vi "HB_ReadAISingleChannel.vi"(8 "error in (no error)":errorcluster, 10 "AI Channel":u8 max=7 step=1, 11 "HBDeviceRef":T1) -> (0 "error out":errorcluster, 1 "Raw Voltage":u32, 2 "Scaled Voltage":dbl, 3 "HBDeviceRef":T1)   [LabVIEW 2016]
uses:
  <vilib>/Rock Robotics/WPI/SerialPort/WPI_SerialPortRef.ctl
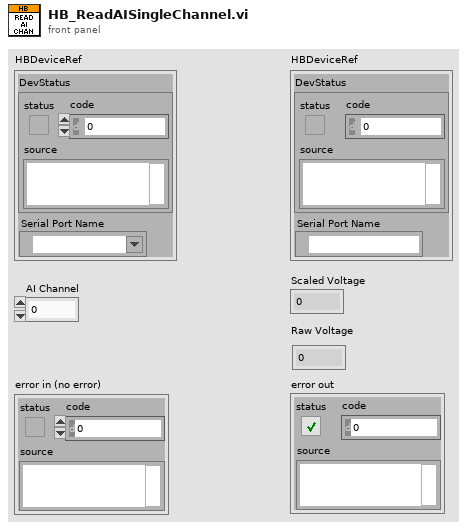
[diagram p1: front panel]
types:
  T1 = typedef "WPI_SerialPortRef.ctl" = cluster{"DevStatus":errorcluster, "Serial Port Name":refnum<visa-resource-name>}
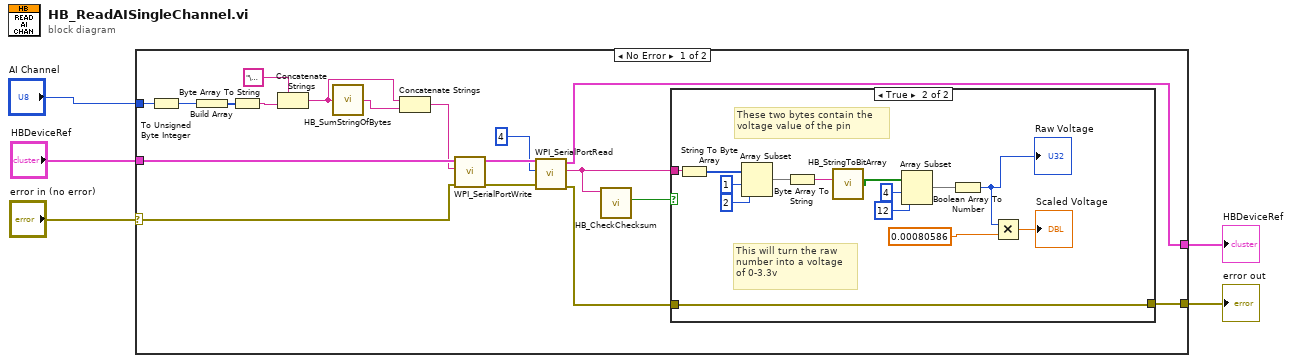
[diagram p0: block diagram]
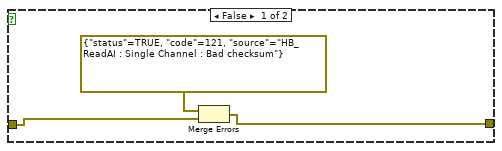
[diagram p2: hidden frame]
diagram:
  n1 = case shown="No Error" "error in (no error)" {
    selector: "error in (no error)" -> [w6 w41]
    tunnel: [w23 w41] -> w5
    tunnel: "HBDeviceRef" -> [w22 w42]
    tunnel: [w21 w42] -> w3
    tunnel: "AI Channel" -> [w7 _]
    frame No Error {
      n2 = To Unsigned Byte Integer(number=w7) -> (unsigned 8bit integer=w14:u8)
      n3 = Build Array(w14) -> (w16:u8[])
      n4 = Byte Array To String(unsigned byte array=w16) -> (string=w12:string)
      n5 = Concatenate Strings("\u0011" ("Buffer"), w12) -> (w9:string)
      n6 = call <vilib>:"HB_SumStringOfBytes.vi"("String Of Bytes"=w9) -> ("Sum as String"=w8:string)
      n7 = Concatenate Strings(w9, w8) -> (w15:string)
      n8 = call <vilib>:"WPI_SerialPortWrite.vi"("error in (no error)"=w6, "Buffer"=w15, "SerialPortRef"=w22) -> ("error out"=w19:errorcluster, "SerialPortRef"=w20:T1)  [unwired: 6 in, 1 out]
      n9 = call <vilib>:"WPI_SerialPortRead.vi"("error in (no error)"=w19, "Num Bytes to Read"=u32 4, "SerialPortRef"=w20) -> ("error out"=w17:errorcluster, "Buffer"=w11:string, "SerialPortRef"=w21:T1)  [unwired: 6 in]
      n10 = call <vilib>:"HB_CheckChecksum.vi"("String"=w11) -> ("Checksum Matches"=w10:bool)  [unwired: 9 in, 1 out]
      n11 = case shown="True" w10 {
        tunnel: w11 -> [_ w30]
        tunnel: w17 -> [w26 w29]
        tunnel: [w24 w29] -> w23
        frame False {
          n12 = Merge Errors(errorcluster {"status"=TRUE, "code"=121, "source"="HB_ReadAI : Single Channel : Bad checksum"} ("error in"), w26) -> (w24:errorcluster)
        }
        frame True {
          # "This will turn the raw \nnumber into a voltage \nof 0-3.3v"
          # "These two bytes contain the \nvoltage value of the pin"
          n13 = String To Byte Array(string=w30) -> (unsigned byte array=w40:u8[])
          n14 = Array Subset(array=w40, index=1, length=2) -> (w37:u8[])
          n15 = Byte Array To String(unsigned byte array=w37) -> (string=w28:string)
          n16 = call <vilib>:"HB_StringToBitArray.vi"("String"=w28) -> ("Bit Array"=w27:bool[])
          n17 = Array Subset(array=w27, index=4, length=12) -> (w34:bool[])
          n18 = Boolean Array To Number(Boolean array=w34) -> (number=w33:u32)
          "Raw Voltage" <- w33
          n19 = Multiply(x=w33, y=0.00080586) -> (x*y=→"Scaled Voltage":dbl)
        }
      }
    }
    frame Error {
    }
  }
  "error out" <- w5
  "HBDeviceRef" <- w3
